vi "Read Readable.vi"(8 "error in (no error)":errorcluster, 11 "Reader.lvclass in":refnum<class "Reader.lvclass">) -> (0 "error out":errorcluster, 2 "Readable.lvclass":refnum<class "Readable.lvclass">, 3 "Reader.lvclass out":refnum<class "Reader.lvclass">)   [LabVIEW 2009, in "Reader.lvclass"]
doc: "(Protected) Return the Readable object associated with this Reader instance, to allow direct manipulation of that Instrument."
uses:
  Reader.lvclass
  Instruments/Utility Classes/Readable/Readable.lvclass
  Reader.lvclass/Reader.ctl
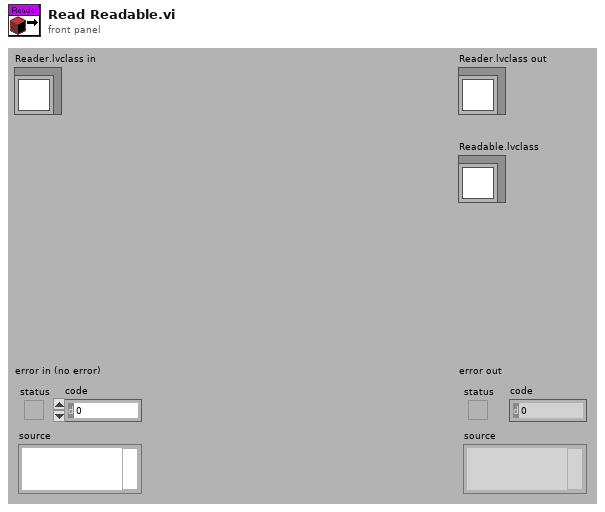
[diagram p1: front panel]
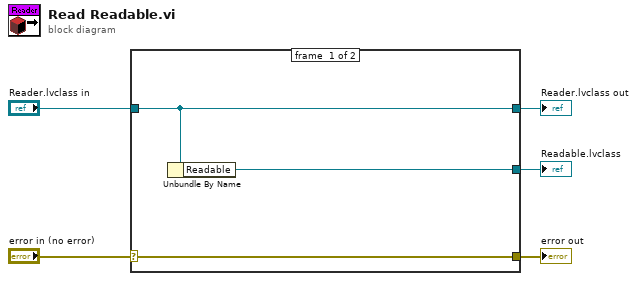
[diagram p0: block diagram]
diagram:
  n1 = case shown="No Error" "error in (no error)" {
    selector: "error in (no error)" -> [w8 w9]
    tunnel: [w8 w9] -> w4
    tunnel: [w7 w10] -> w2
    tunnel: "Reader.lvclass in" -> [w7 w10]
    tunnel: [w6 _] -> w1
    frame #0 {
      n2 = Unbundle By Name(w7) -> ("Readable"=w6:refnum<class "Readable.lvclass">)
    }
    frame #1 {
    }
  }
  "error out" <- w4
  "Reader.lvclass out" <- w2
  "Readable.lvclass" <- w1
